vi "STAT2 decode Digital data from Pressure node.vi"(10 "Pressure Node Data":T2 {"sys register" format="%04x"}) -> (2 "Digital Data Out":T1[](array[typedef]))   [LabVIEW 2011]
uses:
  LEINmaster/Nodes/pressure stat2.ctl
  Measurments Handling/Status Digitalish.ctl
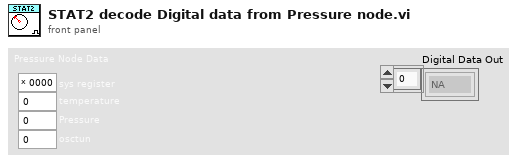
[diagram p1: front panel]
types:
  T1 = typedef "Status Digitalish.ctl" = enum16{"NA", "False", "True"}
  T2 = typedef "pressure stat2.ctl" = cluster{"sys register":u16, "temperature":u16, "Pressure":u16, "osctun":u8}
  T3 = typedef "Stat2 system error.ctl" = cluster{"Error":bool, "Has had error":bool, "Com. issue":bool}
  T4 = typedef "Stat2 system task info.ctl" = cluster{"Task":bool, "Task error":bool, "Task cnt.":u8, "Job 0":bool, "User":bool}
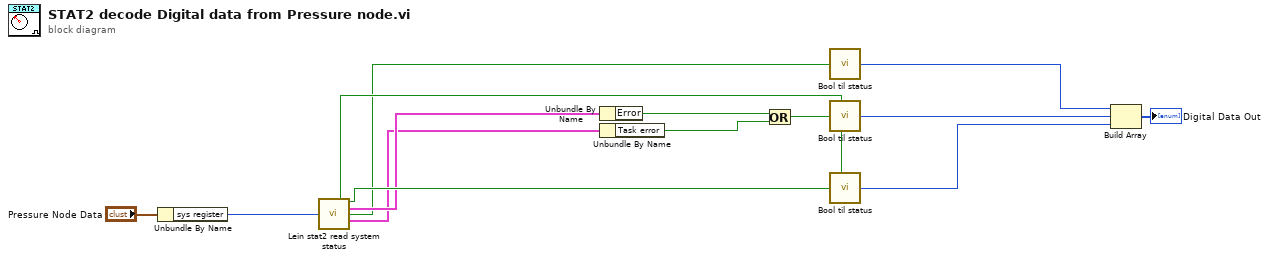
[diagram p0: block diagram]
diagram:
  n1 = Unbundle By Name("Pressure Node Data") -> ("sys register"=w14:u16)
  n2 = call "Lein stat2 read system status.vi"("sys register"=w14) -> ("Force NA"=w7:bool, "Stopped"=w13:bool, "Error"=w9:T3, "Connected"=w5:bool, "Task"=w8:T4)  [unwired: 7 in, 3 out]
  n3 = Unbundle By Name(w9) -> ("Error"=w10:bool)
  n4 = Unbundle By Name(w8) -> ("Task error"=w12:bool)
  n5 = Or(x=w10, y=w12) -> (x .or. y?=w11:bool)
  n6 = call "Bool til status.vi"("Boolean"=w5) -> ("Status"=w4:T1)  [unwired: 8 in]
  n7 = call "Bool til status.vi"("Force NA(F)"=w7, "Boolean"=w11) -> ("Status"=w2:T1)  [unwired: 7 in]
  n8 = call "Bool til status.vi"("Force NA(F)"=w7, "Boolean"=w13) -> ("Status"=w3:T1)  [unwired: 7 in]
  n9 = Build Array(w4, w2, w3) -> (→"Digital Data Out":T1[])
